vi "GetInstance.vi"(8 "error in (no error)":errorcluster, 11 "Registry in":refnum<data-value>) -> (0 "error out":errorcluster, 2 "Instance":refnum<class "NameRegistry.lvclass">, 3 "Registry out":refnum<data-value>)   [LabVIEW 2014, in "UniqueName.lvlib" / "NameRegistry.lvclass"]
uses:
  NameRegistry.lvclass
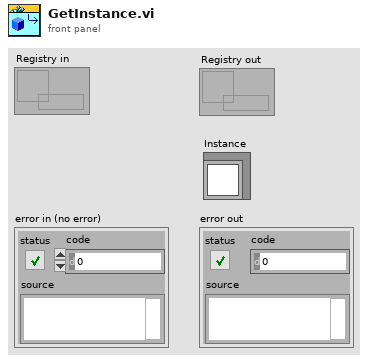
[diagram p1: front panel]
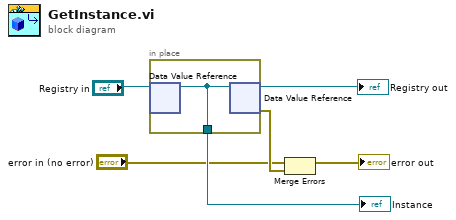
[diagram p0: block diagram]
diagram:
  n1 = in-place {
    in-place-border: [w7] -> w6
    n2 = in-place-dvr #1("Registry in") -> (w7:refnum<class "NameRegistry.lvclass">)  [unwired: 1 out]
    n3 = in-place-dvr #1(w7) -> (→"Registry out":refnum<data-value>, w5:errorcluster)
  }
  "Instance" <- w6
  n4 = Merge Errors("error in (no error)", w5) -> (→"error out":errorcluster)
